vi "Down Sample Waveform Data LV2012 NI Verified.vi"(8 "Error in (no error)":errorcluster, 10 "Desired Sampling Rate":dbl=2000.0, 11 "Waveform in":waveform(dbl)) -> (0 "Error Out":errorcluster, 3 "Waveform out":waveform(dbl))   [LabVIEW 2024]
doc: "This VI takes oversampled data and averages the data to downsample to the desired sampling rate. For instance, if data is captured at 2000 Hz for 1 second and the desired sampling rate is 50 Hz, every new data point is the result of averaging 40 data points (from the 2000 Hz data stream)."
panel:
  # "Overview: This VI accepts arrays of waveforms and down samples them \nRequirements: LabVIEW Full Development System 2012 or compatible\nInstructions:\n1. Initialize the Oversampled Values Array\n2. Enter Desired Sampling Rate \n3. Run the VI"
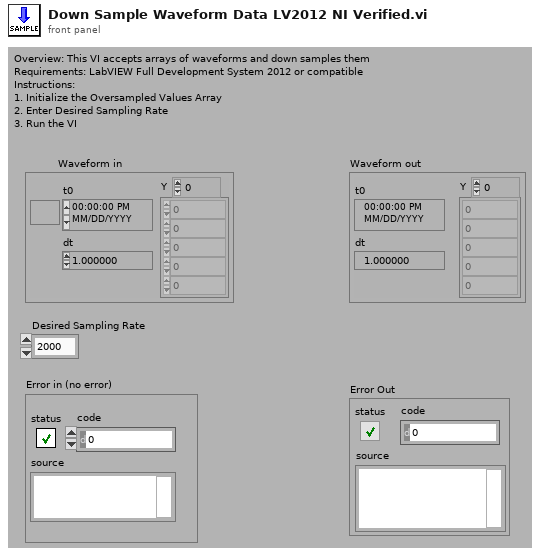
[diagram p1: front panel]
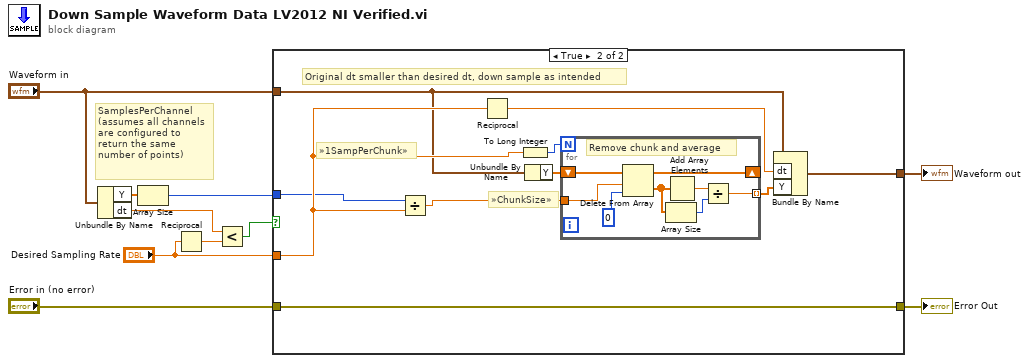
[diagram p0: block diagram]
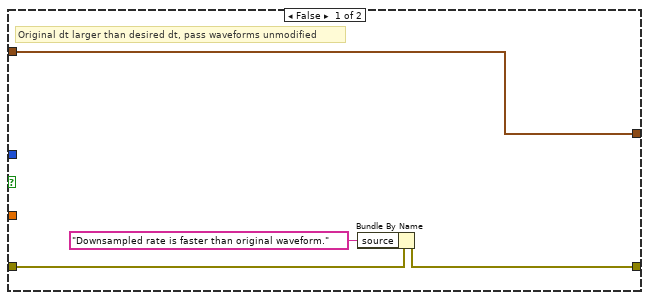
[diagram p2: hidden frame]
diagram:
  # "SamplesPerChannel\n(assumes all channels\nare configured to \nreturn the same \nnumber of points)"
  n1 = Unbundle By Name("Waveform in") -> ("Y"=w10:dbl[], "dt"=w5:dbl)
  n2 = Array Size(array=w10) -> (size(s)=w9:i32)
  n3 = Reciprocal(x="Desired Sampling Rate") -> (1/x=w6:dbl)
  n4 = Less?(x=w5, y=w6) -> (x < y?=w4:bool)
  n5 = case shown="True" w4 {
    tunnel: "Desired Sampling Rate" -> [_ w23]
    tunnel: [w14 w21] -> w2
    tunnel: "Waveform in" -> [w14 w20]
    tunnel: w9 -> [_ w19]
    tunnel: [w12 w18] -> w3
    tunnel: "Error in (no error)" -> [w13 w18]
    frame False {
      # "Original dt larger than desired dt, pass waveforms unmodified"
      n6 = Bundle By Name(cluster=w13, "source"="Downsampled rate is faster than original waveform.") -> (w12:errorcluster)
    }
    frame True {
      # "»ChunkSize»"
      # "Original dt smaller than desired dt, down sample as intended"
      # "»1SampPerChunk»"
      n7 = Divide(x=w19, y=w23) -> (x/y=w24:dbl)
      n8 = Reciprocal(x=w23) -> (1/x=w22:dbl)
      n9 = To Long Integer(number=w23) -> (32bit integer=w15:i32)
      n10 = Unbundle By Name(w20) -> ("Y"=w17:dbl[])
      n11 = for {
        N: w15 -> [_]
        tunnel: [w32] -> w16 mode=indexing
        shift-right: [w28] -> _
        shift-left: w17 -> [w29]
        tunnel: w24 -> [w27]
        # "Remove chunk and average"
        n12 = Delete From Array(array=w29, length=w27, index=0) -> (deleted portion=w26:dbl[], array with subset deleted=w28:dbl[])
        n13 = Array Size(array=w26) -> (size(s)=w25:i32)
        n14 = Add Array Elements(numeric array=w26) -> (sum=w31:dbl)
        n15 = Divide(x=w31, y=w25) -> (x/y=w32:dbl)
      }
      n16 = Bundle By Name(cluster=w20, "dt"=w22, "Y"=w16) -> (w21:waveform(dbl))
    }
  }
  "Error Out" <- w3
  "Waveform out" <- w2
